vi "Scale.vi"() -> ()   [LabVIEW 2018]
panel:
  in  "Normalized Input":dbl
  out "Scaled Output":dbl
  in  "Min":dbl
  in  "Max":dbl
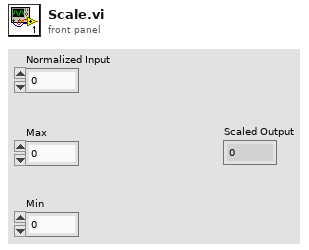
[diagram p1: front panel]
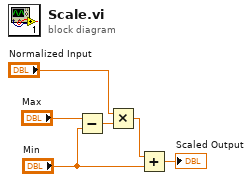
[diagram p0: block diagram]
diagram:
  n1 = Subtract(x="Max", y="Min") -> (x-y=w4:dbl)
  n2 = Multiply(x="Normalized Input", y=w4) -> (x*y=w5:dbl)
  n3 = Add(x=w5, y="Min") -> (x+y=→"Scaled Output":dbl)
